vi "Fetch Measurement (Carrier Frequency Data).vi"(8 "error in (no error)":errorcluster, 11 "VISA resource name":refnum<visa-resource-name>) -> (0 "error out":errorcluster, 2 "Measured Values":dbl[](array[numeric]) format="%#.6g", 3 "VISA resource name out":refnum<visa-resource-name>)   [LabVIEW 2014, in "Agilent ESA PSA Series.lvlib"]
doc: "Returns the results of the last measurement (Carrier Frequency Data) and does not initiate data acquisition.\n\n<B>Note:</B>\n\nThis VI is only valid for the Spot Frequency functionality of the Phase noise personality."
uses:
  Agilent ESA PSA Series.lvlib
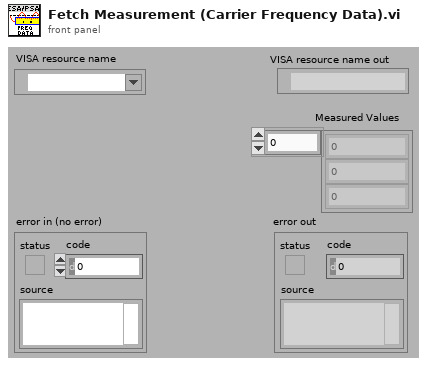
[diagram p1: front panel]
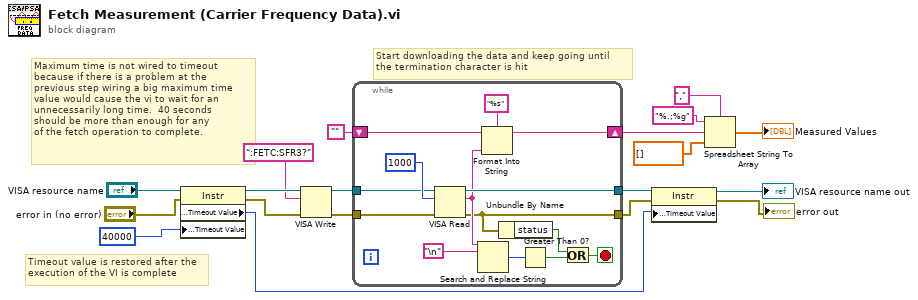
[diagram p0: block diagram]
diagram:
  # "Maximum time is not wired to timeout\nbecause if there is a problem at the\nprevious step wiring a big maximum time\nvalue would cause the vi to wait for an\nunnecessarily long time.  40 seconds\nshould be more than enough for any\nof the fetch operation to complete."
  # "Timeout value is restored after the\nexecution of the VI is complete"
  # "Start downloading the data and keep going until\nthe termination character is hit"
  n1 = property on="Property Node" class="Instr"(reference="VISA resource name", error in="error in (no error)", "General Settings:Timeout Value"=u32 40000) -> (reference out=w16:refnum<visa-resource-name>, error out=w17:errorcluster, "General Settings:Timeout Value"=w13:u32)
  n2 = VISA Write(VISA resource name=w16, write buffer=":FETC:SFR3?", error in (no error)=w17) -> (VISA resource name out=w6:refnum<visa-resource-name>, error out=w5:errorcluster)  [unwired: 1 out]
  n3 = while {
    tunnel: [w32] -> w15
    tunnel: [w20] -> w14
    tunnel: w6 -> [w31]
    tunnel: w5 -> [w30]
    shift-right: [w26] -> w3
    shift-left: "" -> [w25]
    stop <- w22 stop-if-true
    n4 = VISA Read(VISA resource name=w31, byte count=u32 1000, error in (no error)=w30) -> (VISA resource name out=w32:refnum<visa-resource-name>, read buffer=w27:string, error out=w20:errorcluster)  [unwired: 1 out]
    n5 = Search and Replace String(input string=w27, search string="\n") -> (number of replacements=w28:i32)  [unwired: 6 in, 3 out]
    n6 = Format Into String(format string="%s", initial string=w25, w27) -> (resulting string=w26:string)  [unwired: 1 in, 1 out]
    n7 = Unbundle By Name(w20) -> ("status"=w23:bool)
    n8 = Greater Than 0?(x=w28) -> (x > 0?=w21:bool)
    n9 = Or(x=w23, y=w21) -> (x .or. y?=w22:bool)
  }
  n10 = property on="Property Node" class="Instr"(reference=w15, error in=w14, "General Settings:Timeout Value"=w13) -> (reference out=→"VISA resource name out":refnum<visa-resource-name>, error out=→"error out":errorcluster)
  n11 = Spreadsheet String To Array(delimiter (Tab)=",", format string="%.;%g", spreadsheet string=w3, array type (2D Dbl)=dbl[] []) -> (array=→"Measured Values":dbl[])
